vi "Get Number FKV Shift Speeds.vi"(8 "error in (no error)":errorcluster, 11 "number":i32) -> (0 "error out":errorcluster, 2 "function return":u32, 3 "number out":i32)   [LabVIEW 2014, in "atmcd32d.lvlib"]
doc: "unsigned int WINAPI GetNumberFKVShiftSpeeds(int * number);"
uses:
  atmcd32d.lvlib
  atmcd32d.dll
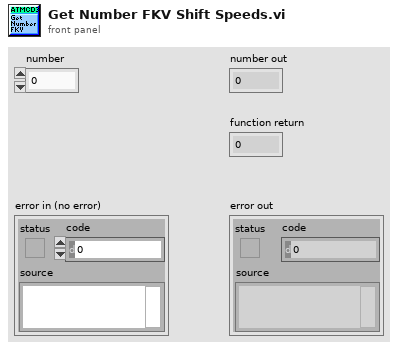
[diagram p1: front panel]
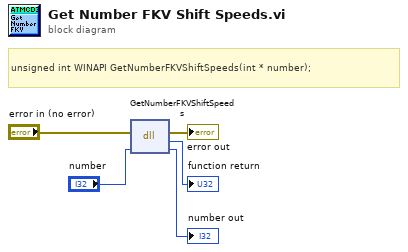
[diagram p0: block diagram]
diagram:
  # "unsigned int WINAPI GetNumberFKVShiftSpeeds(int * number);"
  n1 = dll-call lib="C:/Users/Bakir/Documents/Lambda2-Testing/lib/Andorlib/atmcd32d.*" fn="GetNumberFKVShiftSpeeds"(error in="error in (no error)", "number"="number") -> (error out=→"error out":errorcluster, →"function return":u32, "number"=→"number out":i32)  [unwired: 2 in, 1 out]
